vi "SetSerializeSliceClass.vi"(8 "error in (no error)":errorcluster, 11 "BlueSerializable in":refnum<class "BlueSerializable.lvclass">) -> (0 "error out":errorcluster, 2 "Slice-To-This Class Name":string)   [LabVIEW 2020, in "BlueSerialization.lvlib" / "BlueSerializable.lvclass"]
uses:
  BlueSerializable.lvclass
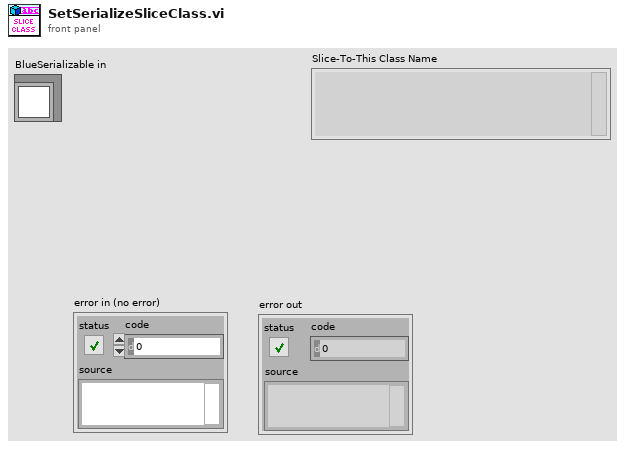
[diagram p1: front panel]
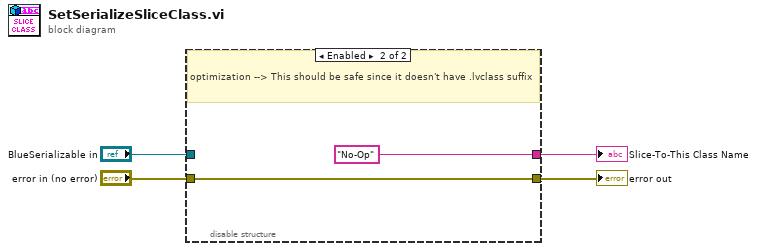
[diagram p0: block diagram]
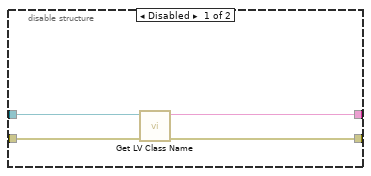
[diagram p2: hidden frame]
diagram:
  n1 = disable-structure shown="Enabled" {
    disable-tunnel: "BlueSerializable in" -> [w8 _]
    disable-tunnel: [w7 "No-Op" ("Slice-To-This Class Name")] -> w3
    disable-tunnel: "error in (no error)" -> [w6 w10]
    disable-tunnel: [w5 w10] -> w1
    frame Disabled {
      n2 = call <vilib>:"Get LV Class Name.vi"("error in (no error)"=w6, "object"=w8) -> ("error out"=w5:errorcluster, "class name"=w7:string)  [unwired: 8 in]
    }
    frame Enabled {
      # "optimization --> This should be safe since it doesn't have .lvclass suffix"
    }
  }
  "Slice-To-This Class Name" <- w3
  "error out" <- w1
